vi "Basic MQTT Publish.vi"() -> ()   [LabVIEW 2017]
uses:
  Demo/Serializer.JKI-JSON/Serializer.JKI-JSON.lvclass
  C:/Program Files (x86)/National Instruments/LabVIEW 2017/vi.lib/LabVIEW Open Source Project/Serializer/Serializer/Serializer.lvclass
  <vilib>/LabVIEW Open Source Project/MQTT Broker/MQTT_Base/MQTT_Base.lvclass/MQTT_Base.ctl
  <vilib>/LabVIEW Open Source Project/MQTT Broker/Client/Client.lvclass/Client.ctl
  <vilib>/LabVIEW Open Source Project/MQTT Broker/Control Packets/ControlPacket/QualityOfService -- enum.ctl
  <vilib>/LabVIEW Open Source Project/MQTT Broker/Client/Client.lvclass
  C:/Program Files (x86)/National Instruments/LabVIEW 2017/vi.lib/LabVIEW Open Source Project/MQTT Broker/MQTT_Base/MQTT_Base.lvclass
  <vilib>/LabVIEW Open Source Project/Serializer/Serializer.FlattenedString/Serializer.FlattenedString.lvclass
  <vilib>/LabVIEW Open Source Project/Serializer/Serializer/Serializer.lvclass
  <vilib>/LabVIEW Open Source Project/MQTT Broker/Control Packets/PUBLISH/PUBLISH.lvclass
  <vilib>/LabVIEW Open Source Project/MQTT Broker/MQTT_Base/MQTT_Base.lvclass
  <vilib>/LabVIEW Open Source Project/MQTT Broker/Control Packets/ControlPacket/ControlPacket.lvclass
panel:
  in  "Anything":variant
  out "error out":errorcluster
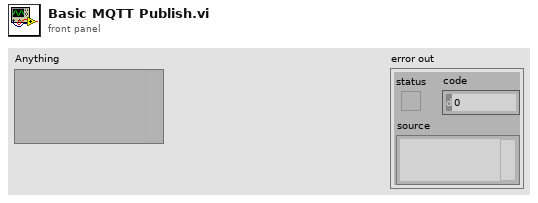
[diagram p1: front panel]
types:
  T1 = typedef "MQTT Server.lvlib/Client.lvclass/Public Events -- cluster.ctl" = cluster{"Connection Status":refnum<user-event>, "Connected":refnum<user-event>, "Application Message":refnum<user-event>}
  T2 = typedef "ControlPacket.lvclass/QualityOfService -- enum.ctl" = enum16{"0 (At Most Once)", "1 (At Least Once)", "2 (Exactly Once)"}
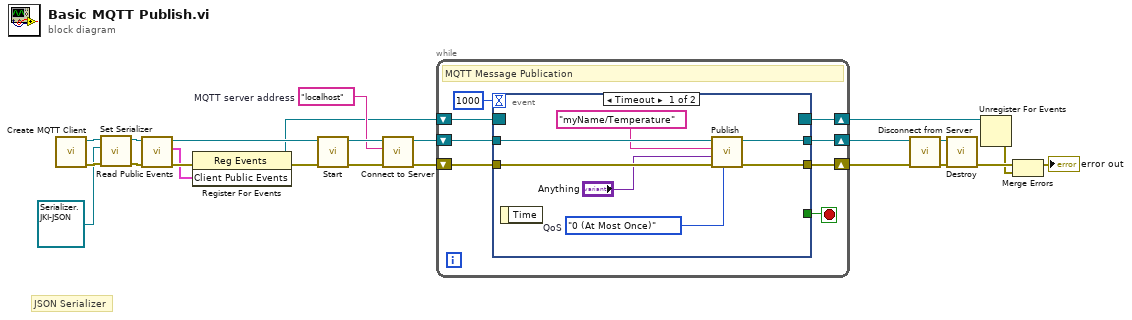
[diagram p0: block diagram]
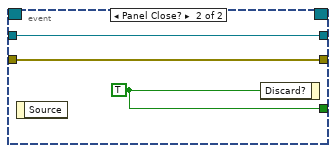
[diagram p2: hidden frame]
diagram:
  w17 = "localhost"  # MQTT server address
  # "JSON Serializer"
  n1 = call <vilib>:"Create MQTT Client.vi"() -> ("error out"=w3:errorcluster, "Client out"=w5:refnum<class "Client.lvclass">)  [unwired: 10 in]
  n2 = call <vilib>:"Set Serializer.vi"("error in (no error)"=w3, "Serializer (default: Flattened String)"=refnum<class "Serializer.JKI-JSON.lvclass"> refnum ("Serializer.JKI-JSON.lvclass"), "MQTT_Base"=w5) -> ("error out"=w2:errorcluster, "MQTT_Base out"=w4:refnum<class "Client.lvclass">)  [unwired: 7 in]
  n3 = call <vilib>:"Read Public Events.vi"("error in (no error)"=w2, "Client in"=w4) -> ("error out"=w20:errorcluster, "Client Public Events"=w18:T1, "Client out"=w21:refnum<class "Client.lvclass">)  [unwired: 7 in]
  n4 = register-events(error in=w20, w18) -> (reference out=w14:refnum<event-registration>, error out=w19:errorcluster)  [unwired: 1 in]
  n5 = call <vilib>:"Start.vi"("error in (no error)"=w19, "MQTT_Base in"=w21) -> ("error out"=w22:errorcluster, "MQTT_Base out"=w23:refnum<class "Client.lvclass">)  [unwired: 7 in, 1 out]
  n6 = call <vilib>:"Connect to Server.vi"("error in (no error)"=w22, "address (localhost)"=w17, "Client in"=w23) -> ("error out"=w8:errorcluster, "Client out"=w9:refnum<class "Client.lvclass">)  [unwired: 5 in, 2 out]
  n7 = while {
    shift-right: [w28] -> w7
    shift-left: w9 -> [w30]
    shift-right: [w27] -> w6
    shift-left: w8 -> [w29]
    shift-right: [w24] -> w13
    shift-left: w14 -> [w25]
    stop <- w26 stop-if-true
    # "MQTT Message Publication"
    n8 = event shown="[0] Timeout" {
      selector: w25 -> [_ _]
      dyn-events: [_ _] -> w24
      timeout: 1000 -> [_ _]
      tunnel: w30 -> [w38 w41]
      tunnel: w29 -> [w36 w40]
      tunnel: [w37 w41] -> w28
      tunnel: [w35 w40] -> w27
      tunnel: [_ w39] -> w26
      event Timeout {
        w32 = QualityOfService_--_enum."0 (At Most Once)"  # QoS
        n9 = event-data() -> ()  [unwired: 1 in, 1 out]
        n10 = call <vilib>:"Publish.vi"("QoS"=w32, "error in (no error)"=w36, "Payload"="Anything", "Topic Name (empty: Payload name)"="myName/Temperature", "Client in"=w38) -> ("error out"=w35:errorcluster, "Client out"=w37:refnum<class "Client.lvclass">)  [unwired: 4 in, 1 out]
      }
      event Panel Close? {
        w39 = TRUE ("Discard?")
        n11 = event-data() -> ()  [unwired: 1 in, 1 out]
        n12 = event-data("Discard?"=w39) -> ()  [unwired: 1 in, 1 out]
      }
    }
  }
  n13 = call <vilib>:"Disconnect from Server.vi"("error in (no error)"=w6, "Client in"=w7) -> ("error out"=w16:errorcluster, "Client out"=w15:refnum<class "Client.lvclass">)  [unwired: 7 in, 1 out]
  n14 = call-dynamic "Destroy.vi"("error in (no error)"=w16, "MQTT_Base in"=w15) -> ("error out"=w12:errorcluster)  [unwired: 8 in, 1 out]
  n15 = Unregister For Events(event registration refnum=w13) -> (error out=w10:errorcluster)  [unwired: 1 in]
  n16 = Merge Errors(w12, w10) -> (→"error out":errorcluster)
